vi "Scan from String.vi"(8 "error in (no error)":errorcluster, 11 "read buffer":string) -> (0 "error out":errorcluster, 2 "Cryostat Temp (K)":dbl, 3 "Sample Stage (K)":dbl)   [LabVIEW 2019]
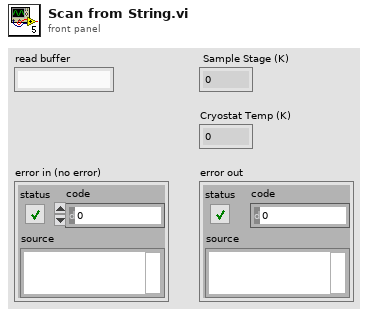
[diagram p1: front panel]
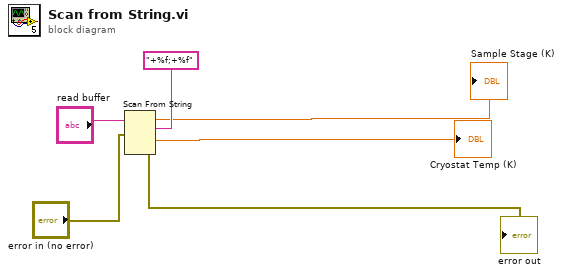
[diagram p0: block diagram]
diagram:
  n1 = Scan From String(format string="+%f;+%f", input string="read buffer", error in="error in (no error)") -> (error out=→"error out":errorcluster, output 1=→"Sample Stage (K)":dbl, output 2=→"Cryostat Temp (K)":dbl)  [unwired: 3 in, 2 out]
